vi "Init.vi"(5 "Project Path":path=path "\\\\vmware-host\\Shared Folders/_Repo/DAQ-Waveform-Function-Generator-Custom-Device/Source/Waveform Analog Output Custom Device.lvproj", 7 "Working Directory":path=path "\\\\vmware-host\\Shared Folders/_Repo/DAQ-Waveform-Function-Generator-Custom-Device/Release", 9 "Version":u32=2020, 11 "error in (no error)":errorcluster) -> (4 "Package Builder out":refnum<class "Package Builder.lvclass">, 15 "error out":errorcluster)   [LabVIEW 2020, in "Package Builder.lvclass"]
uses:
  Package Builder.lvclass
  Package Builder.lvclass/Package Builder.ctl
  Shared/Shared.lvlib
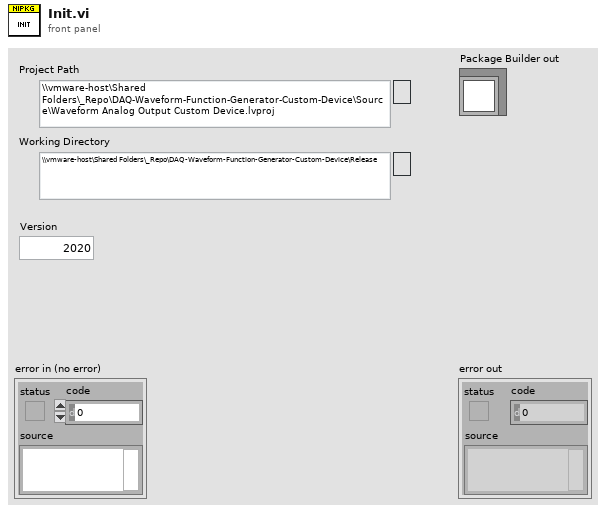
[diagram p1: front panel]
types:
  T1 = enum16{"open", "replace", "create", "open or create", "replace or create", "replace or create with confirmation"}
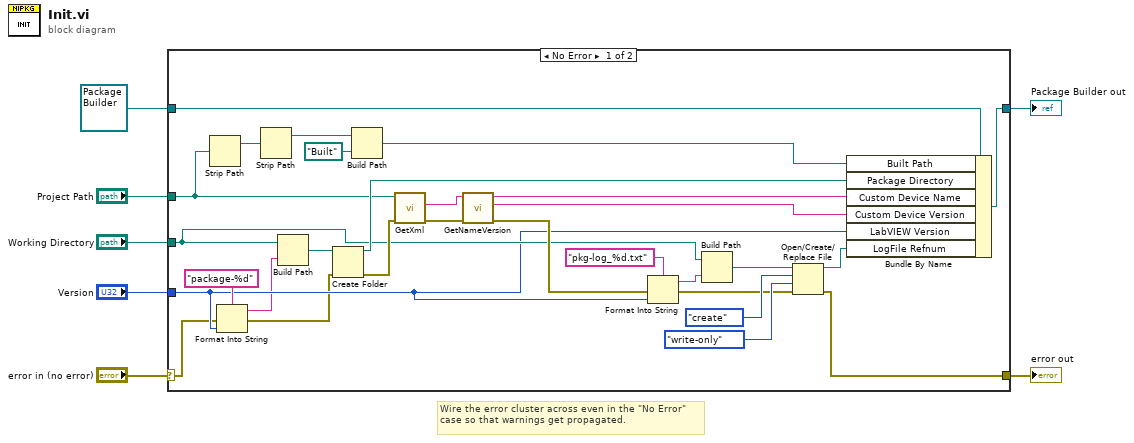
[diagram p0: block diagram]
diagram:
  # "Wire the error cluster across even in the \"No Error\"\ncase so that warnings get propagated."
  n1 = case shown="No Error" "error in (no error)" {
    selector: "error in (no error)" -> [w11 w38]
    tunnel: [w15 w38] -> w6
    tunnel: [w35 w37] -> w4
    tunnel: refnum<class "Package Builder.lvclass"> refnum ("Package Builder in") -> [w36 w37]
    tunnel: "Working Directory" -> [w17 _]
    tunnel: "Project Path" -> [w29 _]
    tunnel: "Version" -> [w12 _]
    frame No Error {
      n2 = Strip Path(path=w29) -> (stripped path=w28:path)  [unwired: 1 out]
      n3 = Format Into String(format string="package-%d", error in=w11, w12) -> (resulting string=w9:string, error out=w10:errorcluster)  [unwired: 1 in]
      n4 = Strip Path(path=w28) -> (stripped path=w27:path)  [unwired: 1 out]
      n5 = Build Path(base path=w17, name or relative path=w9) -> (appended path=w14:path)
      n6 = Create Folder(path (use dialog)=w14, error in=w10) -> (created path=w34:path, error out=w33:errorcluster)  [unwired: 1 in, 1 out]
      n7 = Build Path(base path=w27, name or relative path=path "Built") -> (appended path=w26:path)
      n8 = call "GetXml.vi"("error in (no error)"=w33, "Project Path"=w29) -> ("error out"=w30:errorcluster, "XML String"=w8:string)  [unwired: 7 in, 1 out]
      n9 = call "GetNameVersion.vi"("error in (no error)"=w30, "XML String"=w8) -> ("error out"=w18:errorcluster, "Custom Device Version"=w31:string, "Custom Device Name"=w32:string)  [unwired: 7 in]
      n10 = Format Into String(format string="pkg-log_%d.txt" ("time format string (%c)"), error in=w18, w12) -> (resulting string=w20:string, error out=w21:errorcluster)  [unwired: 1 in]
      n11 = Build Path(base path=w17, name or relative path=w20) -> (appended path=w22:path)
      n12 = Open/Create/Replace File(file path (use dialog)=w22, error in=w21, operation (0:open)=T1."create", access (0:read/write)=enum16{"read/write", "read-only", "write-only"}."write-only") -> (refnum out=w16:refnum<file>, error out=w15:errorcluster)  [unwired: 2 in, 1 out]
      n13 = Bundle By Name(cluster=w36, "Built Path"=w26, "Package Directory"=w34, "Custom Device Name"=w32, "Custom Device Version"=w31, "LabVIEW Version"=w12, "LogFile Refnum"=w16) -> (w35:refnum<class "Package Builder.lvclass">)
    }
    frame Error {
    }
  }
  "error out" <- w6
  "Package Builder out" <- w4
